vi "Is Open Delimiter.vi"(8 "Error In":errorcluster, 11 "Parser In":refnum<class "Parser.lvclass">) -> (0 "Error Out":errorcluster, 2 "Open Delimiter":bool, 3 "Parser Out":refnum<class "Parser.lvclass">)   [LabVIEW 2018, in "Toolkit.lvlib" / "Parser.lvclass"]
uses:
  Parser.lvclass
  Parser.lvclass/Parser.ctl
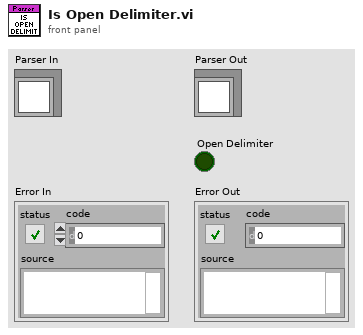
[diagram p1: front panel]
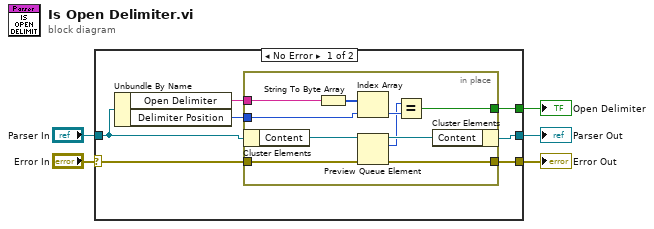
[diagram p0: block diagram]
diagram:
  n1 = case shown="No Error" "Error In" {
    selector: "Error In" -> [w7 w24]
    tunnel: [w6 w24] -> w4
    tunnel: "Parser In" -> [w12 w23]
    tunnel: [w11 w23] -> w2
    tunnel: [w8 _] -> w1
    frame No Error {
      n2 = Unbundle By Name(w12) -> ("Open Delimiter"=w9:string, "Delimiter Position"=w10:i32)
      n3 = in-place {
        in-place-border: w10 -> [w20]
        in-place-border: w9 -> [w19]
        in-place-border: [w18] -> w8
        in-place-border: w7 -> [w14]
        in-place-border: [w13] -> w6
        n4 = in-place-cluster #1(w12) -> ("Content"=w17:refnum<queue>)
        n5 = String To Byte Array(string=w19) -> (unsigned byte array=w21:u8[])
        n6 = Index Array(array=w21, index=w20) -> (element=w22:u8)
        n7 = Preview Queue Element(queue=w17, error in (no error)=w14) -> (queue out=w16:refnum<queue>, element=w15:u8, error out=w13:errorcluster)  [unwired: 1 in, 1 out]
        n8 = Equal?(x=w15, y=w22) -> (x = y?=w18:bool)
        n9 = in-place-cluster #1("Content"=w16) -> (w11:refnum<class "Parser.lvclass">)
      }
    }
    frame Error {
    }
  }
  "Error Out" <- w4
  "Parser Out" <- w2
  "Open Delimiter" <- w1
